vi "SvgDoc Get Fill Color.vi"(8 "error in (no error)":errorcluster, 11 ".NET Refnum in":refnum<k24>) -> (0 "error out":errorcluster, 2 "Color Box":u32(colorbox), 3 "reference out":refnum<k24>)   [LabVIEW 2020, in "SvgDotNet.lvlib"]
uses:
  SvgDotNet.lvlib
  C:/Users/huipeng8/Desktop/SVG.NET/Svg.dll
  Svg.dll
panel:
  out "ToString":string
  # "Connector Pane"
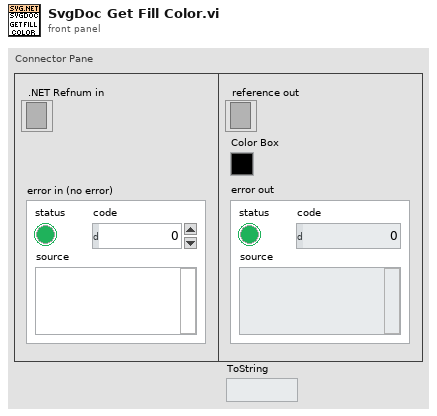
[diagram p1: front panel]
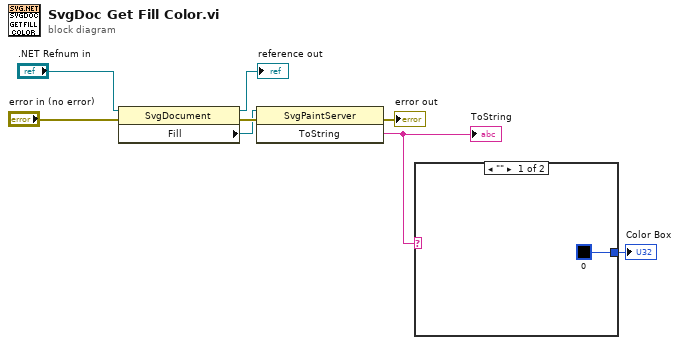
[diagram p0: block diagram]
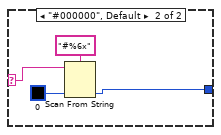
[diagram p2: hidden frame]
diagram:
  n1 = property class="SvgDocument"(reference=".NET Refnum in", error in="error in (no error)") -> (reference out=→"reference out":refnum<k24>, error out=w6:errorcluster, "Fill"=w5:refnum<k24>)
  n2 = invoke class="SvgPaintServer" method="ToString"(reference=w5, error in=w6) -> (error out=→"error out":errorcluster, "ToString"=w2:string)  [unwired: 1 in, 1 out]
  "ToString" <- w2
  n3 = case shown="\"\"" w2 {
    selector: w2 -> [_ w11]
    tunnel: [u32 0 w10] -> w1
    frame "" {
    }
    frame "#000000", Default {
      n4 = Scan From String(format string="#%6x", input string=w11, default 1=u32 0) -> (output 1=w10:u32)  [unwired: 2 in, 3 out]
    }
  }
  "Color Box" <- w1
